vi "sound output.vi"() -> ()   [LabVIEW 2016]
panel:
  in  "设备ID":u32
  out "正在播放声音？":bool
  in  "停止":bool
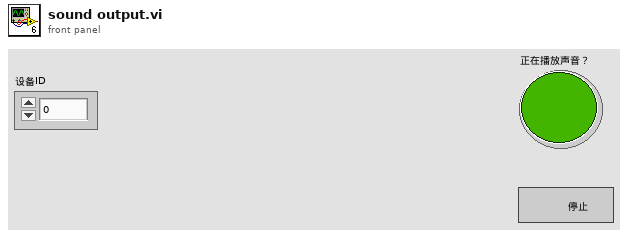
[diagram p1: front panel]
types:
  T1 = typedef "Sound Output Task ID.ctl" = u32
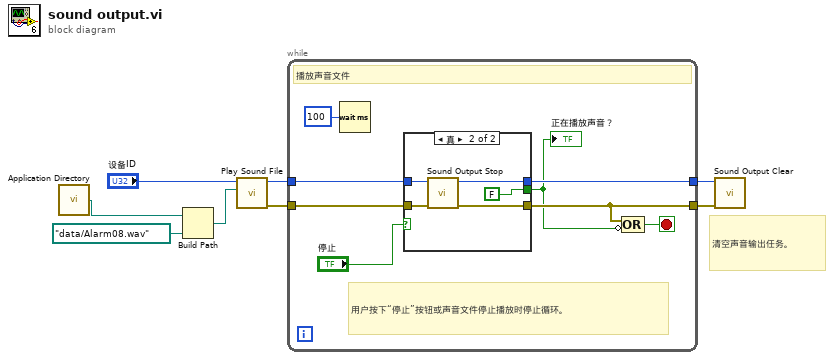
[diagram p0: block diagram]
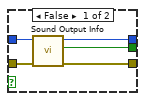
[diagram p2: hidden frame]
diagram:
  # "清空声音输出任务。"
  n1 = call <vilib>:"Application Directory.vi"() -> ("Application Directory"=w1:path)
  n2 = Build Path(base path=w1, name or relative path=path "data/Alarm08.wav" ("Sound File Path")) -> (appended path=w2:path)
  n3 = call <vilib>:"Play Sound File.vi"("path"=w2, "device ID"="设备ID") -> ("error out"=w7:errorcluster, "task ID"=w8:T1)  [unwired: 8 in]
  n4 = while {
    tunnel: w8 -> [w10]
    tunnel: [w15] -> w5
    tunnel: w7 -> [w11]
    tunnel: [w14] -> w6
    stop <- w16 stop-if-true
    # "用户按下“停止”按钮或声音文件停止播放时停止循环。"
    # "播放声音文件"
    n5 = Wait (ms)(milliseconds to wait=u32 100) -> ()  [unwired: 1 out]
    n6 = case shown="真" "停止" {
      tunnel: w11 -> [w21 w25]
      tunnel: [w20 w23] -> w15
      tunnel: w10 -> [w19 w26]
      tunnel: [w18 w24] -> w14
      tunnel: [w17 FALSE] -> w13
      frame False {
        n7 = call <vilib>:"Sound Output Info.vi"("error in (no error)"=w21, "task ID"=w19) -> ("error out"=w18:errorcluster, "is playing?"=w17:bool, "task ID out"=w20:T1)  [unwired: 6 in, 1 out]
      }
      frame True {
        n8 = call <vilib>:"Sound Output Stop.vi"("error in (no error)"=w25, "task ID"=w26) -> ("error out"=w24:errorcluster, "task ID out"=w23:T1)  [unwired: 8 in]
      }
    }
    "正在播放声音？" <- w13
    n9 = Compound Arithmetic op=OR(w14, invert w13) -> (w16:bool)
  }
  n10 = call <vilib>:"Sound Output Clear.vi"("error in (no error)"=w6, "task ID"=w5) -> ()  [unwired: 9 in, 1 out]
